vi "_General_VoltageOutput.vi"() -> ()   [LabVIEW 2012]
uses:
  <vilib>/DAQmx/write.llb/DAQmx Write (Analog 1D DBL NChan 1Samp).vi
  <vilib>/DAQmx/miscellaneous.llb/DAQmx Fill In Error Info.vi
panel:
  out "Voltages 2":dbl[](array[numeric]) format="%0.2f"
  out "Iteration":i32
  in  "stop":bool
  in  "Voltages":dbl[](array[numeric]) format="%0.2f"
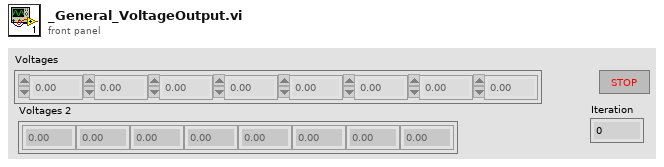
[diagram p1: front panel]
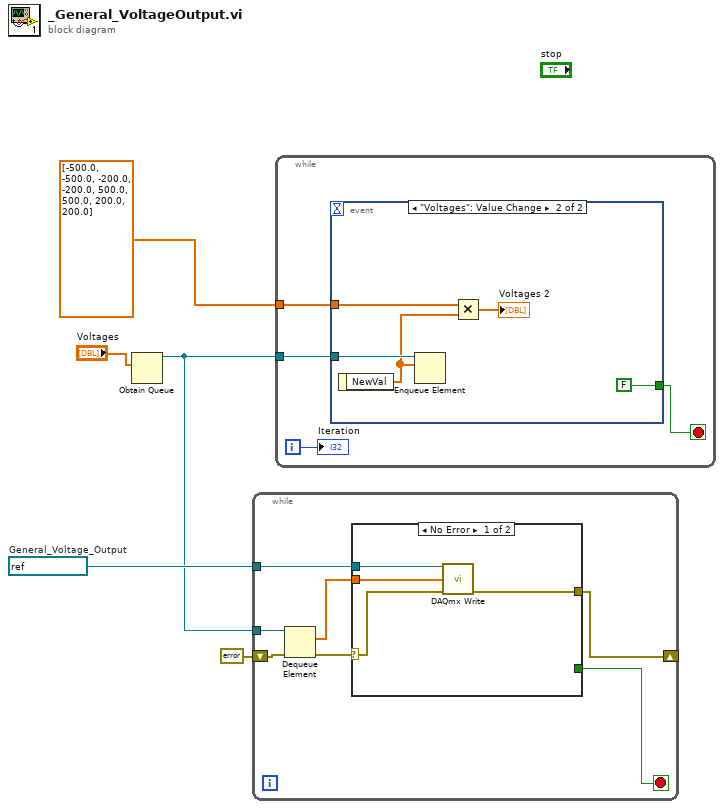
[diagram p0: block diagram]
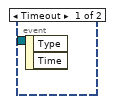
[diagram p2: hidden frame]
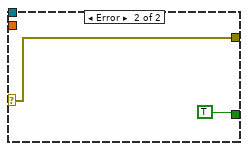
[diagram p3: hidden frame]
diagram:
  w5 = refnum<k21> "Emco_HV"  # General_Voltage_Output
  n1 = Obtain Queue(element data type="Voltages") -> (queue out=w3:refnum<queue>)  [unwired: 4 in, 2 out]
  n2 = while {
    tunnel: w5 -> [w12]
    tunnel: w3 -> [w11]
    shift-right: [w7] -> _
    shift-left: errorcluster {"status"=FALSE, "code"=0, "source"=""} ("error out") -> [w6]
    stop <- w8 stop-if-true
    n3 = Dequeue Element(queue=w11, error in (no error)=w6) -> (element=w10:dbl[], error out=w9:errorcluster)  [unwired: 1 in, 2 out]
    n4 = case shown="No Error" w9 {
      selector: w9 -> [w13 w17]
      tunnel: w12 -> [w16 _]
      tunnel: w10 -> [w15 _]
      tunnel: [_ TRUE] -> w8
      tunnel: [w14 w17] -> w7
      frame No Error {
        n5 = call-poly <vilib>:"DAQmx Write.vi"("task/channels in"=w16, "data"=w15, "error in"=w13) -> ("error out"=w14:errorcluster)  [unwired: 10 in, 2 out]
      }
      frame Error {
      }
    }
  }
  n6 = while {
    tunnel: w3 -> [w22]
    tunnel: dbl[] [-500.0, -500.0, -200.0, -200.0, 500.0, 500.0, 200.0, 200.0] ("x") -> [w19]
    i -> [w20]
    stop <- w21 stop-if-true
    n7 = event shown="[1] \"Voltages\": Value Change" {
      selector: _ -> [_ _]
      dyn-events: _ -> [_ _]
      timeout: _ -> [_ _]
      tunnel: w22 -> [_ w27]
      tunnel: [_ FALSE] -> w21
      tunnel: w19 -> [_ w23]
      event Timeout {
        n8 = event-data() -> ()  [unwired: 1 in, 2 out]
      }
      event "Voltages": Value Change {
        n9 = event-data() -> ("NewVal"=w24:dbl[])  [unwired: 1 in]
        n10 = Enqueue Element(queue=w27, element=w24) -> ()  [unwired: 2 in, 3 out]
        n11 = Multiply(x=w23, y=w24) -> (x*y=→"Voltages 2":dbl[])
      }
    }
    "Iteration" <- w20
  }
